vi "Initialize VIs Communication.vi"(8 "error in (no error)":errorcluster, 11 "Channel in":refnum<class "Channel.lvclass">) -> (0 "error out":errorcluster, 3 "Channel out":refnum<class "Channel.lvclass">)   [LabVIEW 2018, in "Channel.lvclass"]
doc: "Initialze the communcation with S4GUI"
uses:
  Channel.lvclass
  Channel.lvclass/Channel.ctl
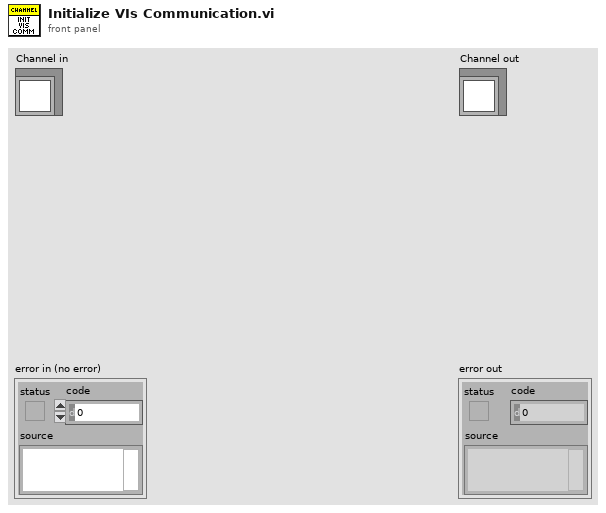
[diagram p1: front panel]
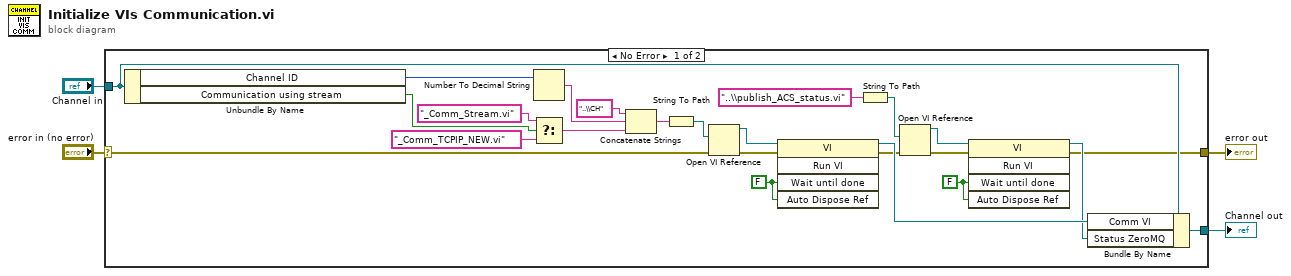
[diagram p0: block diagram]
diagram:
  n1 = case shown="No Error" "error in (no error)" {
    selector: "error in (no error)" -> [w23 w30]
    tunnel: [w7 w30] -> w3
    tunnel: [w14 w29] -> w1
    tunnel: "Channel in" -> [w16 w29]
    frame No Error {
      w10 = FALSE ("Wait Until Done")
      w27 = FALSE ("Wait Until Done")
      n2 = Unbundle By Name(w16) -> ("Channel ID"=w20:u8, "Communication using stream"=w13:bool)
      n3 = Number To Decimal String(number=w20) -> (decimal integer string=w21:string)  [unwired: 1 in]
      n4 = Select(t="_Comm_Stream.vi" ("name or relative path"), s=w13, f="_Comm_TCPIP_NEW.vi" ("name or relative path")) -> (s? t:f=w19:string)
      n5 = Concatenate Strings("..\\CH" ("name or relative path"), w21, w19) -> (w25:string)
      n6 = String To Path(string=w25) -> (path=w26:path)
      n7 = Open VI Reference(vi path=w26, error in (no error)=w23) -> (vi reference=w28:refnum<vi>, error out=w24:errorcluster)  [unwired: 4 in]
      n8 = invoke class="VI" method="Run VI"(reference=w28, error in=w24, "Wait until done"=w27, "Auto Dispose Ref"=w27) -> (reference out=w15:refnum<vi>, error out=w6:errorcluster)  [unwired: 1 in, 3 out]
      n9 = String To Path(string="..\\publish_ACS_status.vi" ("name or relative path")) -> (path=w11:path)
      n10 = Open VI Reference(vi path=w11, error in (no error)=w6) -> (vi reference=w9:refnum<vi>, error out=w12:errorcluster)  [unwired: 4 in]
      n11 = invoke class="VI" method="Run VI"(reference=w9, error in=w12, "Wait until done"=w10, "Auto Dispose Ref"=w10) -> (reference out=w8:refnum<vi>, error out=w7:errorcluster)  [unwired: 1 in, 3 out]
      n12 = Bundle By Name(cluster=w16, "Comm VI"=w15, "Status ZeroMQ"=w8) -> (w14:refnum<class "Channel.lvclass">)
    }
    frame Error {
    }
  }
  "error out" <- w3
  "Channel out" <- w1
